vi "TrajectoryExecuteAbsoluteInterrupt.vi"(7 "command":string, 8 "Init":bool, 9 "commandstarttime":dbl, 10 "End Abs\nOrientation Deg":dbl, 11 "Trajectory":T1 {"States"."POSE"."ROTATION"."SIN" format="%13.4f"; "States"."POSE"."ROTATION"."COS" format="%13.4f"; "States"."POSE"."ROTATION"."VALUE" format="%13.4f"; "States"."POSE"."TRANSLATION"."Y" format="%14.3f"; "States"."POSE"."TRANSLATION"."X" format="%14.3f"; "TotalTImeSecs" format="%20.3f"}) -> (0 "AtReference":bool, 3 "Chassis Velocity Target":T6 {"vOmega" format="%10.3f"; "vY" format="%10.3f"; "vX" format="%10.3f"})   [LabVIEW 2023]
uses:
  <vilib>/Rock Robotics/WPI/ThirdParty/JAS_Junk/TrajLib/TypeDef/CHASSIS_SPEEDS.ctl
  <vilib>/Rock Robotics/WPI/ThirdParty/JAS_Junk/TrajLib/TypeDef/TRAJECTORY.ctl
  <vilib>/Rock Robotics/WPI/ThirdParty/JAS_Junk/TrajLib/TypeDef/TRAJ_STATE.ctl
  <vilib>/Rock Robotics/WPI/ThirdParty/JAS_Junk/TrajLib/TypeDef/POSE2D.ctl
  <vilib>/Rock Robotics/WPI/ThirdParty/JAS_Junk/TrajLib/TypeDef/TRANSLATION2D.ctl
  <vilib>/Rock Robotics/WPI/ThirdParty/JAS_Junk/TrajLib/TypeDef/ROTATION2D.ctl
  <vilib>/Rock Robotics/WPI/ThirdParty/JAS_Junk/TrajLib/PIDController_Pack_Tuning.vi
  <vilib>/Rock Robotics/WPI/ThirdParty/JAS_Junk/TrajLib/HolDrvCtrl_PackProfPID.vi
  <vilib>/Rock Robotics/WPI/ThirdParty/JAS_Junk/TrajLib/VI/HolDrvCtrl_PackControllers.vi
  <vilib>/Rock Robotics/WPI/ThirdParty/JAS_Junk/TrajLib/Pose2d_New.vi
  <vilib>/Rock Robotics/WPI/ThirdParty/JAS_Junk/TrajLib/VI/Util_GetTime_U32.vi
  <vilib>/Rock Robotics/WPI/ThirdParty/JAS_Junk/TrajLib/HolDrvCtrl_New.vi
  <vilib>/Rock Robotics/WPI/ThirdParty/JAS_Junk/TrajLib/HolDrvCtrl_PackPID.vi
  <vilib>/Rock Robotics/WPI/ThirdParty/JAS_Junk/TrajLib/HolDrvCtrl_SetTolerance.vi
  <vilib>/Rock Robotics/WPI/ThirdParty/JAS_Junk/TrajLib/HolDrvCtrl_SetEnabled.vi
  <vilib>/Rock Robotics/WPI/ThirdParty/JAS_Junk/TrajLib/HolDrvCtrl_Calculate_Trajectory.vi
  <vilib>/Rock Robotics/WPI/ThirdParty/JAS_Junk/TrajLib/HolDrvCtrl_AtReference.vi
  <vilib>/Rock Robotics/WPI/ThirdParty/JAS_Junk/TrajLib/ProfiledPIDController_NewPeriod.vi
  <vilib>/Rock Robotics/WPI/ThirdParty/JAS_Junk/TrajLib/ProfiledPIDController_SetIntegratorRange.vi
  <vilib>/Rock Robotics/WPI/ThirdParty/JAS_Junk/TrajLib/ProfiledPIDController_DisableContInput.vi
  <vilib>/Rock Robotics/WPI/ThirdParty/JAS_Junk/TrajLib/ProfiledPIDController_EnableContInput.vi
  <vilib>/Rock Robotics/WPI/ThirdParty/JAS_Junk/TrajLib/TrapProfConstraint_New.vi
  <vilib>/Rock Robotics/WPI/ThirdParty/JAS_Junk/TrajLib/Rotation2d_CreateAngle.vi
  <vilib>/Rock Robotics/WPI/ThirdParty/JAS_Junk/TrajLib/Translation2d_Create.vi
  <vilib>/Rock Robotics/WPI/ThirdParty/JAS_Junk/TrajLib/Conv_Deg_Radians.vi
  <vilib>/Rock Robotics/WPI/ThirdParty/JAS_Junk/TrajLib/PIDController_NewPeriod.vi
  <vilib>/Rock Robotics/WPI/ThirdParty/JAS_Junk/TrajLib/PIDController_SetIntegratorRange.vi
  <vilib>/Rock Robotics/WPI/ThirdParty/JAS_Junk/TrajLib/PIDController_Reset.vi
  <vilib>/Rock Robotics/WPI/ThirdParty/JAS_Junk/TrajLib/HolDrvCtrl_Calculate.vi
  <vilib>/Rock Robotics/WPI/ThirdParty/JAS_Junk/TrajLib/Rotation2d_GetRadians.vi
  <vilib>/Rock Robotics/WPI/ThirdParty/JAS_Junk/TrajLib/TrapProfState_New.vi
  <vilib>/Rock Robotics/SystemInterfaces/NetworkCommunication/NetComm_UsageReport_report.vi
  <vilib>/Rock Robotics/WPI/ThirdParty/JAS_Junk/TrajLib/PIDController_DisableContinousInput.vi
  <vilib>/Rock Robotics/WPI/ThirdParty/JAS_Junk/TrajLib/PIDController_EnableContinousInput.vi
  <vilib>/Rock Robotics/WPI/ThirdParty/JAS_Junk/TrajLib/Rotation2d_GetAngleCosSin.vi
  <vilib>/Rock Robotics/WPI/ThirdParty/JAS_Junk/TrajLib/Pose2d_RelativeTo.vi
  <vilib>/Rock Robotics/WPI/ThirdParty/JAS_Junk/TrajLib/Pose2d_getRotation.vi
  <vilib>/Rock Robotics/WPI/ThirdParty/JAS_Junk/TrajLib/Rotation2d_Minus.vi
  <vilib>/Rock Robotics/WPI/ThirdParty/JAS_Junk/TrajLib/ProfiledPIDController_Calculate_Meas_Goal.vi
  <vilib>/Rock Robotics/WPI/ThirdParty/JAS_Junk/TrajLib/PIDController_Calculate_SP_PV.vi
  <vilib>/Rock Robotics/WPI/ThirdParty/JAS_Junk/TrajLib/ProfiledPIDController_Reset_PosOnly.vi
  <vilib>/Rock Robotics/WPI/ThirdParty/JAS_Junk/TrajLib/ChassisSpeeds_FromFieldRelativeSpeeds.vi
  <vilib>/Rock Robotics/WPI/ThirdParty/JAS_Junk/TrajLib/Transform2d_Create_PosePose.vi
  <vilib>/Rock Robotics/WPI/ThirdParty/JAS_Junk/TrajLib/Pose2d_New_TRRO.vi
  <vilib>/Rock Robotics/WPI/ThirdParty/JAS_Junk/TrajLib/Rotation2d_UnaryMinus.vi
  <vilib>/Rock Robotics/WPI/ThirdParty/JAS_Junk/TrajLib/Rotation2d_RotateBy.vi
  <vilib>/Rock Robotics/WPI/ThirdParty/JAS_Junk/TrajLib/ProfiledPIDController_SetGoal_PosOnly.vi
  <vilib>/Rock Robotics/WPI/ThirdParty/JAS_Junk/TrajLib/ProfiledPIDController_Calculate_Meas.vi
  <vilib>/Rock Robotics/WPI/ThirdParty/JAS_Junk/TrajLib/PIDController_SetSetpoint.vi
  <vilib>/Rock Robotics/WPI/ThirdParty/JAS_Junk/TrajLib/PIDController_Calculate_PV.vi
  <vilib>/Rock Robotics/WPI/ThirdParty/JAS_Junk/TrajLib/ProfiledPIDController_Reset.vi
  <vilib>/Rock Robotics/WPI/ThirdParty/JAS_Junk/TrajLib/Rotation2d_GetCos.vi
  <vilib>/Rock Robotics/WPI/ThirdParty/JAS_Junk/TrajLib/Rotation2d_GetSin.vi
  <vilib>/Rock Robotics/WPI/ThirdParty/JAS_Junk/TrajLib/Translation2d_RotateBy.vi
  <vilib>/Rock Robotics/WPI/ThirdParty/JAS_Junk/TrajLib/Translation2d_Minus.vi
  <vilib>/Rock Robotics/WPI/ThirdParty/JAS_Junk/TrajLib/Rotation2d_CreateXY.vi
  <vilib>/Rock Robotics/WPI/ThirdParty/JAS_Junk/TrajLib/ProfiledPIDController_SetGoal.vi
  <vilib>/Rock Robotics/WPI/ThirdParty/JAS_Junk/TrajLib/TrapProfile_New.vi
  <vilib>/Rock Robotics/WPI/ThirdParty/JAS_Junk/TrajLib/ProfiledPIDController_GetPeriod.vi
  <vilib>/Rock Robotics/WPI/ThirdParty/JAS_Junk/TrajLib/TrapProfile_Calculate.vi
  <vilib>/Rock Robotics/WPI/ThirdParty/JAS_Junk/TrajLib/ControllerUtil_GetModulusError.vi
  <vilib>/Rock Robotics/WPI/ThirdParty/JAS_Junk/TrajLib/Util_CalcDist.vi
  <vilib>/Rock Robotics/WPI/ThirdParty/JAS_Junk/TrajLib/TrapProfile_ShouldFlipAcceleration.vi
  <vilib>/Rock Robotics/WPI/ThirdParty/JAS_Junk/TrajLib/TrapProfile_Direct.vi
  <vilib>/Rock Robotics/WPI/ThirdParty/JAS_Junk/TrajLib/PIDController_GetPeriod.vi
  <vilib>/Rock Robotics/WPI/ThirdParty/JAS_Junk/TrajLib/VI/Util_GetTime_U64.vi
  TrajectoryGlobals.vi
  Vision/VisionGlobal.vi
  <vilib>/Rock Robotics/WPI/ThirdParty/JAS_Junk/TrajLib/Globals/Util_LibraryGlobals.vi
  <vilib>/Rock Robotics/WPI/ThirdParty/JAS_Junk/TrajLib/Trajectory_Library.lvlib
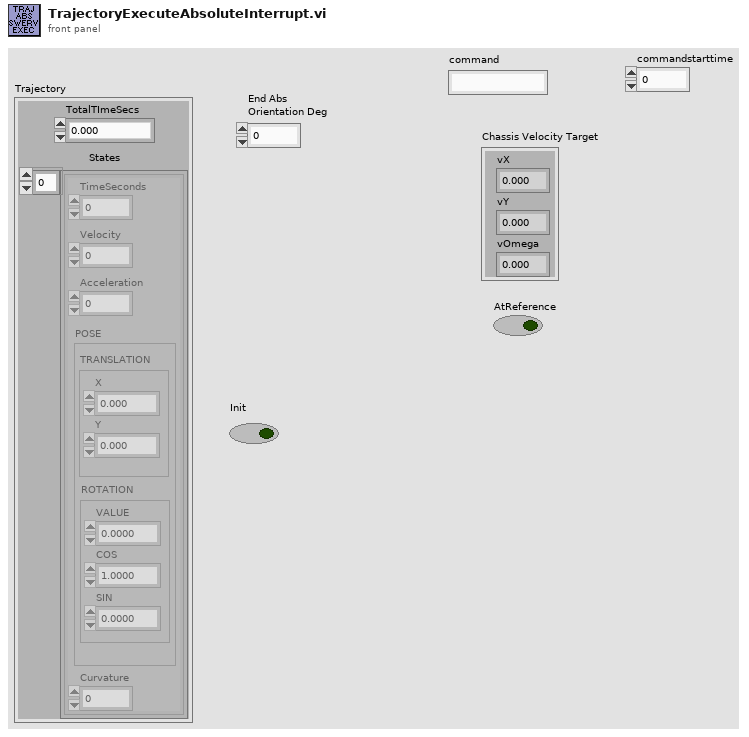
[diagram p1: front panel]
types:
  T1 = typedef "Trajectory_Library.lvlib/TRAJECTORY.ctl" = cluster{"TotalTImeSecs":dbl, "States":T2[]}
  T2 = typedef "Trajectory_Library.lvlib/TRAJ_STATE.ctl" = cluster{"TimeSeconds":dbl, "Velocity":dbl, "Acceleration":dbl, "POSE":T3, "Curvature":dbl}
  T3 = typedef "Trajectory_Library.lvlib/POSE2D.ctl" = cluster{"TRANSLATION":T4, "ROTATION":T5}
  T4 = typedef "Trajectory_Library.lvlib/TRANSLATION2D.ctl" = cluster{"X":dbl, "Y":dbl}
  T5 = typedef "Trajectory_Library.lvlib/ROTATION2D.ctl" = cluster{"VALUE":dbl, "COS":dbl, "SIN":dbl}
  T6 = typedef "Trajectory_Library.lvlib/CHASSIS_SPEEDS.ctl" = cluster{"vX":dbl, "vY":dbl, "vOmega":dbl}
  T7 = typedef "Trajectory_Library.lvlib/HOLONOMIC_PACK_TUNING.ctl" = cluster{"X PID Tuning":T8, "Y PID Tuning":T8, "thetaProfiledPID_CTRL":T9}
  T8 = typedef "Trajectory_Library.lvlib/PID_TUNING.ctl" = cluster{"Kp":dbl, "Ki":dbl, "Kd":dbl, "MaximumIntegral":dbl, "MinimumIntegral":dbl, "IntegralZone":dbl}
  T9 = typedef "Trajectory_Library.lvlib/PROFILED_PID_CONTROLLER.ctl" = cluster{"Controller":T10, "Goal":T11, "Setpoint":T11, "Constraint":T12}
  T10 = typedef "Trajectory_Library.lvlib/PID_CONTROLLER.ctl" = cluster{"Kp":dbl, "Ki":dbl, "Kd":dbl, "Period":dbl, "Max_Integral":dbl, "Min_Integral":dbl, "Max_Input":dbl, "Min_Input":dbl, "Continuous":bool, "PositionError":dbl, "VelocityError":dbl, "PrevError":dbl, "Total_Integral":dbl, "PositionTolerance":dbl, "VelocityTolerance":dbl, "SetPoint":dbl, "Kf":dbl, "Prev_Deriv":dbl, "Prev_Deriv 2":dbl, "DerivativeFilter":bool, "Min_Output":dbl, "Max_Output":dbl, "Prev_F_P":dbl, "Prev_F_P_2":dbl, "AntiWindupActive":bool, "Measurement":dbl, "IntegralZone":dbl}
  T11 = typedef "Trajectory_Library.lvlib/TRAPEZOID_PROFILE_STATE.ctl" = cluster{"Position":dbl, "Velocity":dbl}
  T12 = typedef "Trajectory_Library.lvlib/TRAPEZOID_PROFILE_CONSTRAINT.ctl" = cluster{"MaxVelocity":dbl, "MaxAcceleration":dbl}
  T13 = typedef "Trajectory_Library.lvlib/HOLONOMIC_DRV_CTRL.ctl" = cluster{"poseTolerance":T3, "poseError":T3, "Enabled":bool, "PID_xCtrl":T10, "PID_yCtrl":T10, "PROF_PID_thetaCtrl":T9, "RotationError":T5, "FirstRun":bool}
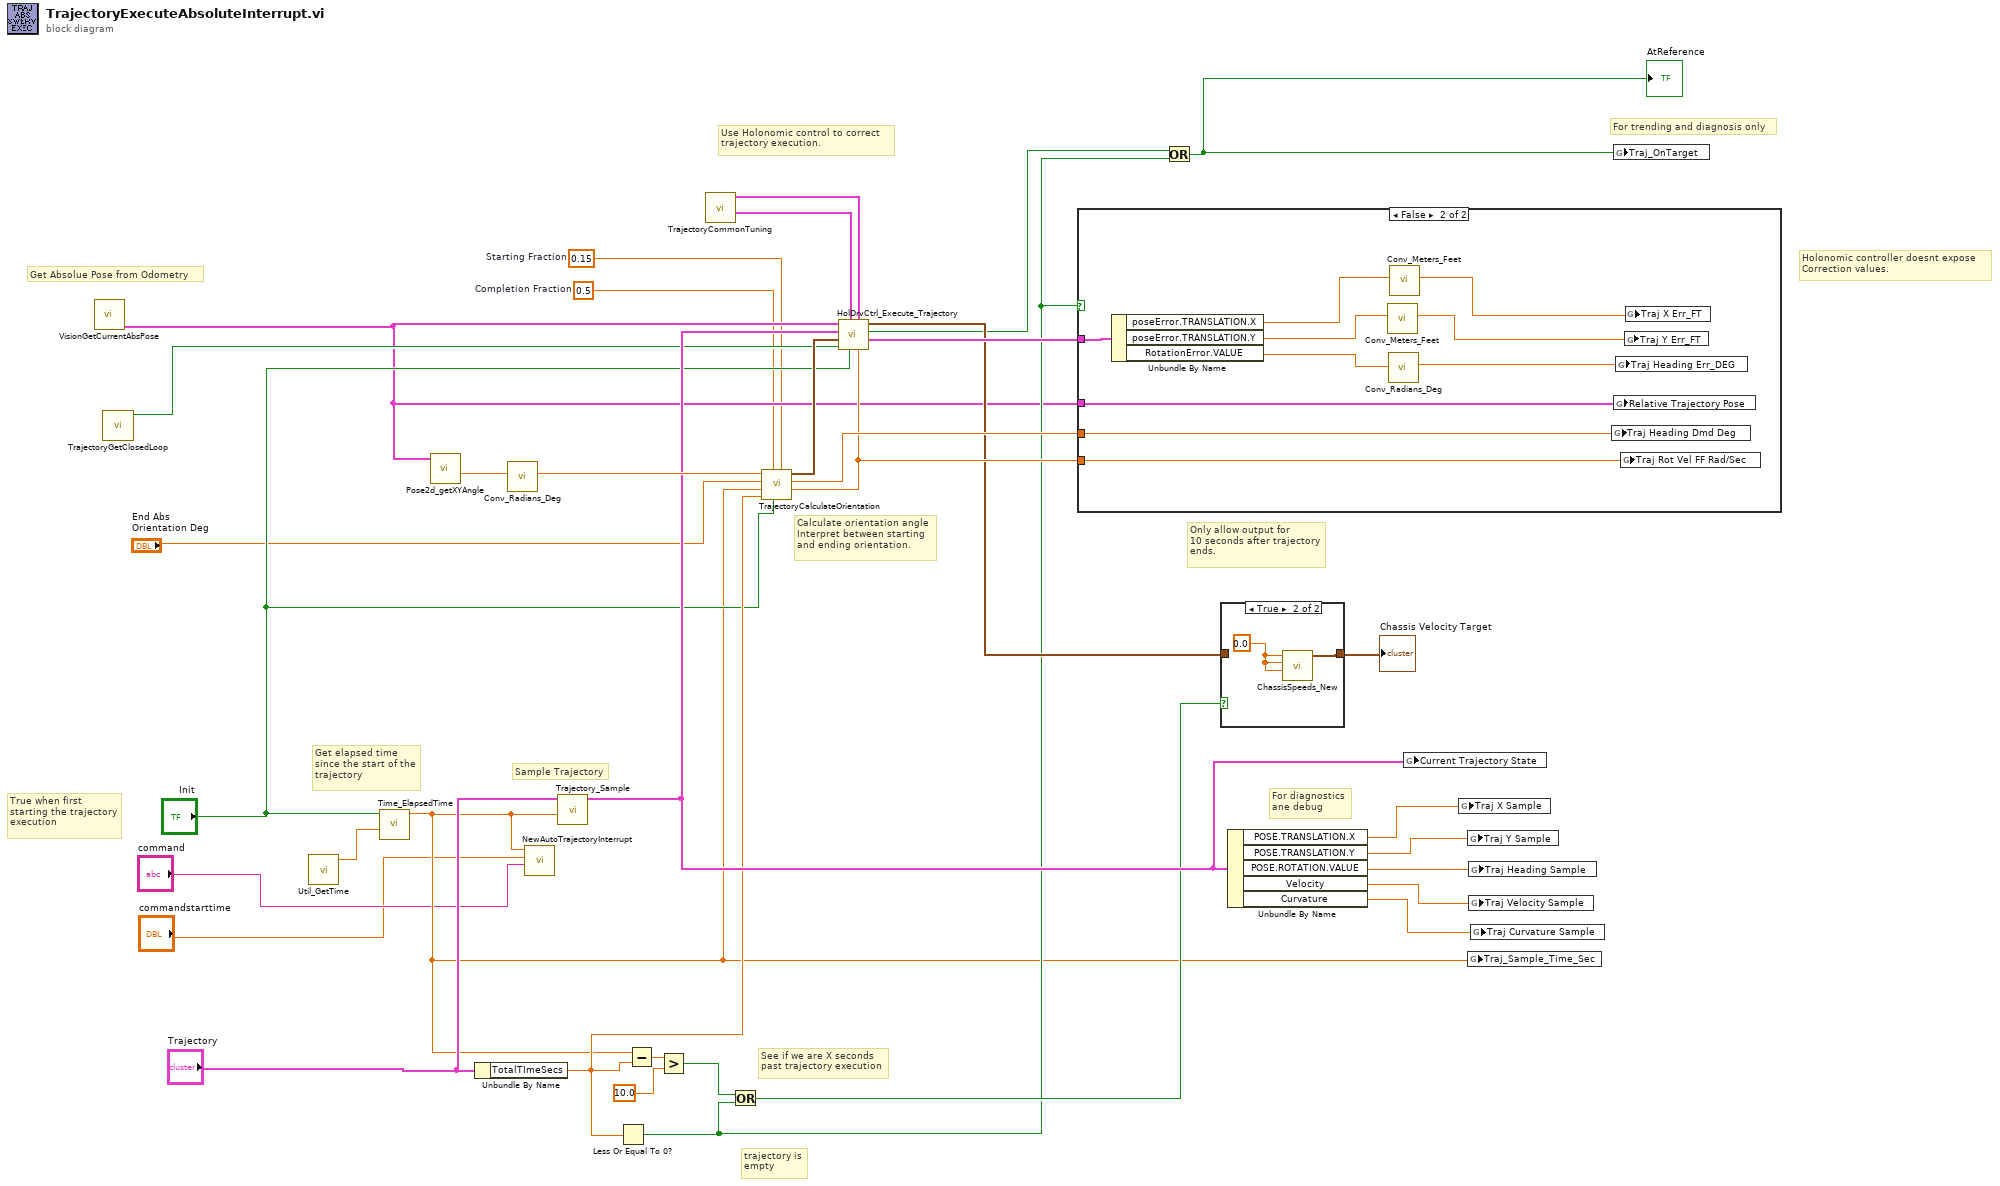
[diagram p0: block diagram]
diagram:
  w6 = 0.15  # Starting Fraction
  w7 = 0.5  # Completion Fraction
  # "trajectory is \nempty"
  # "Calculate orientation angle\nInterpret between starting\nand ending orientation."
  # "True when first\nstarting the trajectory\nexecution"
  # "Get elapsed time\nsince the start of the\ntrajectory"
  # "Holonomic controller doesnt expose\nCorrection values."
  # "Use Holonomic control to correct\ntrajectory execution."
  # "For trending and diagnosis only"
  # "For diagnostics\nane debug"
  # "Get Absolue Pose from Odometry"
  # "Sample Trajectory"
  # "See if we are X seconds \npast trajectory execution"
  # "Only allow output for\n10 seconds after trajectory\nends."
  n1 = call "VisionGetCurrentAbsPose.vi"() -> ("Current ABS Pose"=w10:T3)  [unwired: 9 in]
  n2 = call "TrajectoryGetClosedLoop.vi"() -> ("AUTO_CLOSED_LOOP"=w11:bool)  [unwired: 11 in]
  n3 = call <vilib>:"Util_GetTime.vi"() -> ("FPGA_Time_Seconds"=w32:dbl)  [unwired: 9 in, 2 out]
  n4 = call <vilib>:"Time_ElapsedTime.vi"("PassthroughTime_SEC"=w32, "Reset"="Init") -> ("Elapsed Time Sec"=w3:dbl)  [unwired: 9 in]
  n5 = call <vilib>:"Pose2d_getXYAngle.vi"("in POSE"=w10) -> ("Angle"=w22:dbl)  [unwired: 8 in, 2 out]
  n6 = Unbundle By Name("Trajectory") -> ("TotalTImeSecs"=w13:dbl)
  n7 = call <vilib>:"Conv_Radians_Deg.vi"("Radians"=w22) -> ("Degrees"=w21:dbl)  [unwired: 10 in]
  n8 = call "NewAutoTrajectoryInterrupt.vi"("command"="command", "commandtime"="commandstarttime", "elapsedtime"=w3) -> ()  [unwired: 9 in]
  n9 = call <vilib>:"Trajectory_Sample.vi"("Time"=w3, "InputTRAJECTORY"="Trajectory") -> ("OutputTRAJ_STATE"=w20:T2)  [unwired: 9 in]
  n10 = Less Or Equal To 0?(x=w13) -> (x <= 0?=w14:bool)
  n11 = Subtract(x=w3, y=w13) -> (x-y=w35:dbl)
  n12 = Greater?(x=w35, y=10.0) -> (0:w18:bool)
  n13 = call "TrajectoryCommonTuning.vi"() -> ("out POSe"=w8:T3, "HOLONOMIC_CTRL_PACK_TUNING"=w9:T7)  [unwired: 10 in]
  n14 = Or(x=w18, y=w14) -> (x .or. y?=w17:bool)
  n15 = call "TrajectoryCalculateOrientation.vi"("Starting Fraction"=w6, "Init"="Init", "Completion Fraction"=w7, "Total Trajectory Time Sec"=w13, "Elapsed Traj Time Sec"=w3, "End Orientation Demand DEG"="End Abs\nOrientation Deg", "Starting Orientation  DEG"=w21) -> ("Rotational Velocity Rad Per Sec"=w23:dbl, "Orientation Demand Deg"=w26:dbl, "Orientation Demand"=w25:T5)  [unwired: 2 in]
  n16 = call <vilib>:"HolDrvCtrl_Execute_Trajectory.vi"("Rotational Velocity Feedforward \nRad/Sec"=w23, "HOLONOMIC_CTRL_PACK_TUNING"=w9, "Reset"="Init", "Tolerance"=w8, "Enable"=w11, "angleRef"=w25, "desiredTrajState"=w20, "currentPose"=w10) -> ("outHOLONOMIC_DRV_CTRL"=w24:T13, "AtReference"=w16:bool, "calcChassisSpeed"=w19:T6)  [unwired: 1 in]
  n17 = case shown="False" w14 {
    tunnel: w26 -> [_ w45]
    tunnel: w24 -> [_ w39]
    tunnel: w23 -> [_ w38]
    tunnel: w10 -> [_ w36]
    frame True {
    }
    frame False {
      n18 = Unbundle By Name(w39) -> ("poseError.TRANSLATION.X"=w43:dbl, "poseError.TRANSLATION.Y"=w42:dbl, "RotationError.VALUE"=w37:dbl)
      n19 = call <vilib>:"Conv_Meters_Feet.vi"("Meters"=w42) -> ("Feet"=w41:dbl)  [unwired: 10 in]
      n20 = call <vilib>:"Conv_Radians_Deg.vi"("Radians"=w37) -> ("Degrees"=w44:dbl)  [unwired: 10 in]
      n21 = call <vilib>:"Conv_Meters_Feet.vi"("Meters"=w43) -> ("Feet"=w40:dbl)  [unwired: 10 in]
      n22 = global write "TrajectoryGlobals.vi" "Traj Heading Dmd Deg"(w45) -> ()
      n23 = global write "TrajectoryGlobals.vi" "Relative Trajectory Pose"(w36) -> ()
      n24 = global write "TrajectoryGlobals.vi" "Traj Heading Err_DEG"(w44) -> ()
      n25 = global write "TrajectoryGlobals.vi" "Traj Rot Vel FF Rad/Sec"(w38) -> ()
      n26 = global write "TrajectoryGlobals.vi" "Traj Y Err_FT"(w41) -> ()
      n27 = global write "TrajectoryGlobals.vi" "Traj X Err_FT"(w40) -> ()
    }
  }
  n28 = Or(x=w16, y=w14) -> (x .or. y?=w15:bool)
  "AtReference" <- w15
  n29 = case shown="True" w17 {
    tunnel: w19 -> [w46 _]
    tunnel: [w46 w47] -> w33
    frame False {
    }
    frame True {
      w48 = 0.0 ("vX")
      n30 = call <vilib>:"ChassisSpeeds_New.vi"("vAngular"=w48, "vY"=w48, "vX"=w48) -> ("CHASSIS"=w47:T6)  [unwired: 8 in]
    }
  }
  "Chassis Velocity Target" <- w33
  n31 = Unbundle By Name(w20) -> ("POSE.TRANSLATION.X"=w31:dbl, "POSE.TRANSLATION.Y"=w30:dbl, "POSE.ROTATION.VALUE"=w29:dbl, "Velocity"=w28:dbl, "Curvature"=w27:dbl)
  n32 = global write "TrajectoryGlobals.vi" "Current Trajectory State"(w20) -> ()
  n33 = global write "TrajectoryGlobals.vi" "Traj X Sample"(w31) -> ()
  n34 = global write "TrajectoryGlobals.vi" "Traj Y Sample"(w30) -> ()
  n35 = global write "TrajectoryGlobals.vi" "Traj_Sample_Time_Sec"(w3) -> ()
  n36 = global write "TrajectoryGlobals.vi" "Traj Heading Sample"(w29) -> ()
  n37 = global write "TrajectoryGlobals.vi" "Traj Velocity Sample"(w28) -> ()
  n38 = global write "TrajectoryGlobals.vi" "Traj Curvature Sample"(w27) -> ()
  n39 = global write "TrajectoryGlobals.vi" "Traj_OnTarget"(w15) -> ()
